vi "AnalyzeWithinUncertainty (SubVI).vi"(5 "Uncertainty on mean x":dbl, 7 "Mean x":dbl, 8 "error in (no error)":errorcluster, 9 "y uncertainties":dbl[](array[numeric]), 10 "y values":dbl[](array[numeric]), 11 "x values":dbl[](array[numeric])) -> (0 "error out":errorcluster, 2 "Mean of y uncertainties":dbl, 3 "Mean y":dbl)   [LabVIEW 2016]
uses:
  <vilib>/measure/mascope.llb/Transition Measurements 1 chan.vi
  <vilib>/measure/NI_MAPro.lvlib
panel:
  out "Uncertainty on mean y":dbl
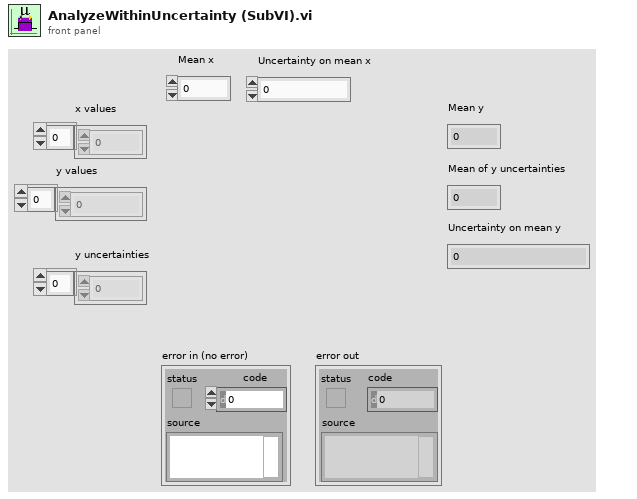
[diagram p1: front panel]
types:
  T1 = cluster{"start time":dbl, "end time":dbl, "ref levels":cluster{"high ref level":dbl, "mid ref level":dbl, "low ref level":dbl, "ref units":u16}}
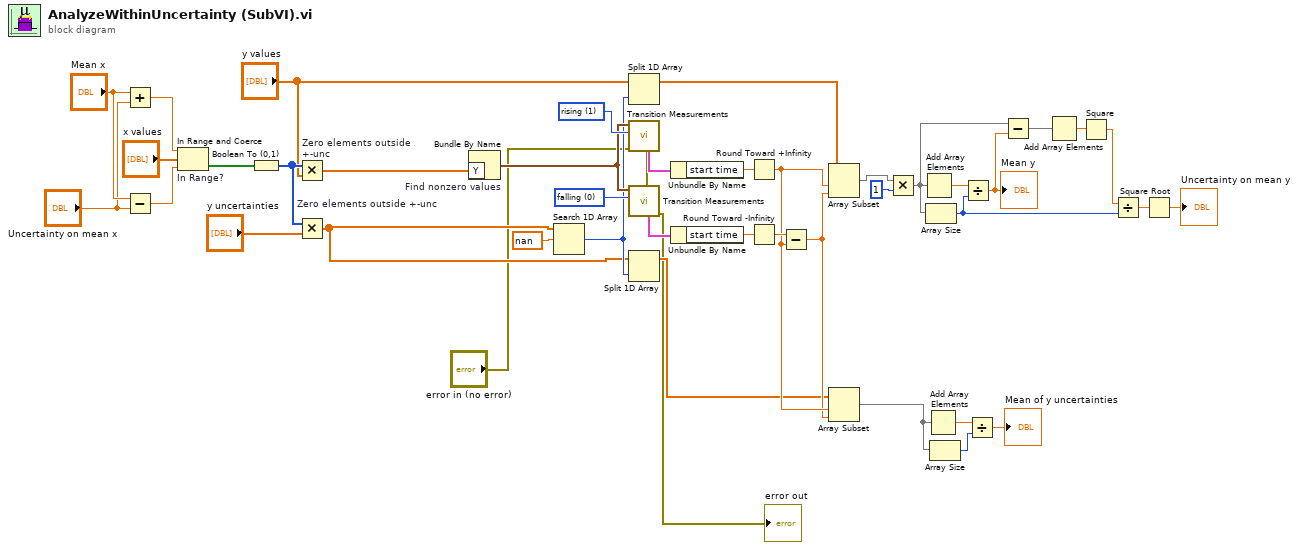
[diagram p0: block diagram]
diagram:
  w42 = u16 1 items=["falling", "rising"] ("polarity (rising)")
  w38 = u16 0 items=["falling", "rising"] ("polarity (rising)")
  n1 = Add(x="Mean x", y="Uncertainty on mean x") -> (x+y=w33:dbl)
  n2 = Subtract(x="Mean x", y="Uncertainty on mean x") -> (x-y=w32:dbl)
  n3 = In Range and Coerce "In Range?"(upper limit=w33, x="x values", lower limit=w32) -> (In Range?=w37:bool[])  [unwired: 1 out]
  n4 = Boolean To (0,1)(Boolean=w37) -> (0, 1=w27:i16[])
  n5 = Multiply "Zero elements outside +-unc"(x=w27, y="y values") -> (x*y=w40:dbl[])
  n6 = Multiply "Zero elements outside +-unc"(x=w27, y="y uncertainties") -> (x*y=w22:dbl[])
  n7 = Bundle By Name "Find nonzero values"("Y"=w40) -> (w41:waveform(dbl))  [unwired: 1 in]
  n8 = Search 1D Array(1D array=w22, element=nan) -> (index of element=w24:i32)  [unwired: 1 in]
  n9 = Split 1D Array(array="y values", index=w24) -> (first subarray=w23:dbl[])  [unwired: 1 out]
  n10 = call-poly <vilib>:"Transition Measurements.vi"("error in (no error)"="error in (no error)", "polarity (rising)"=w42, "signal in"=w41) -> ("error out"=w3:errorcluster, "measurement info"=w43:T1)  [unwired: 3 in, 4 out]
  n11 = call-poly <vilib>:"Transition Measurements.vi"("error in (no error)"=w3, "polarity (rising)"=w38, "signal in"=w41) -> ("error out"=→"error out":errorcluster, "measurement info"=w39:T1)  [unwired: 3 in, 4 out]
  n12 = Split 1D Array(array=w22, index=w24) -> (first subarray=w18:dbl[])  [unwired: 1 out]
  n13 = Unbundle By Name(w43) -> ("start time"=w30:dbl)
  n14 = Unbundle By Name(w39) -> ("start time"=w28:dbl)
  n15 = Round Toward +Infinity(x=w30) -> (ceil(x): smallest int >= x=w21:dbl)
  n16 = Round Toward -Infinity(1:w28) -> (0:w29:dbl)
  n17 = Subtract(x=w29, y=w21) -> (x-y=w20:dbl)
  n18 = Array Subset(array=w23, index=w21, length=w20) -> (w19:dbl[])
  n19 = Array Subset(array=w18, index=w21, length=w20) -> (w4:dbl[])
  n20 = Multiply(x=w19, y=1) -> (x*y=w15:dbl[])
  n21 = Add Array Elements(numeric array=w15) -> (sum=w17:dbl)
  n22 = Array Size(array=w15) -> (size(s)=w12:i32)
  n23 = Add Array Elements(numeric array=w4) -> (sum=w5:dbl)
  n24 = Array Size(array=w4) -> (size(s)=w7:i32)
  n25 = Divide(x=w17, y=w12) -> (x/y=w14:dbl)
  "Mean y" <- w14
  n26 = Divide(x=w5, y=w7) -> (x/y=→"Mean of y uncertainties":dbl)
  n27 = Subtract(x=w15, y=w14) -> (x-y=w13:dbl[])
  n28 = Add Array Elements(numeric array=w13) -> (sum=w11:dbl)
  n29 = Square(x=w11) -> (x^2=w10:dbl)
  n30 = Divide(x=w10, y=w12) -> (x/y=w9:dbl)
  n31 = Square Root(x=w9) -> (sqrt(x)=→"Uncertainty on mean y":dbl)
